vi "My_timer_ramp.vi"(9 "Starting Value":dbl, 10 "Final Value":dbl, 11 "Ramp Time [s]":i32) -> (2 "Elapsed Time (s)":dbl, 3 "Out":dbl)   [LabVIEW 2018]
uses:
  de41b6ff-440a-4791-9191-5ec353d1f62a.vi
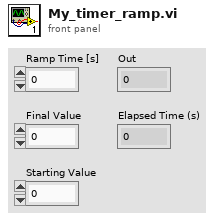
[diagram p1: front panel]
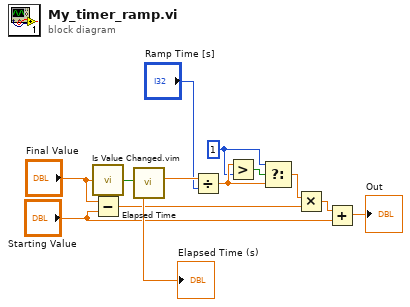
[diagram p0: block diagram]
diagram:
  w9 = 1
  n1 = call "Is Value Changed.vim"("value"="Final Value") -> ("changed or first call?"=w2:bool)
  n2 = Subtract(x="Final Value", y="Starting Value") -> (x-y=w4:dbl)
  n3 = call "Elapsed Time"("Reset"=w2) -> ("Elapsed Time (s)"=w12:dbl)  [unwired: 11 in, 7 out]
  "Elapsed Time (s)" <- w12
  n4 = Divide(x=w12, y="Ramp Time [s]") -> (x/y=w10:dbl)
  n5 = Greater?(x=w10, y=w9) -> (0:w8:bool)
  n6 = Select(t=w9, s=w8, f=w10) -> (s? t:f=w7:dbl)
  n7 = Multiply(x=w7, y=w4) -> (x*y=w6:dbl)
  n8 = Add(x=w6, y="Starting Value") -> (x+y=→"Out":dbl)
